vi "PQsetClientEncoding.vi"(8 "error in (no error)":errorcluster, 10 "encoding":string, 11 "conn":u32) -> (0 "error out":errorcluster, 2 "PQsetClientEncoding":i32)   [LabVIEW 2017, in "libpqlv.lvlib"]
uses:
  libpqlv.lvlib
  lib/libpq.dll
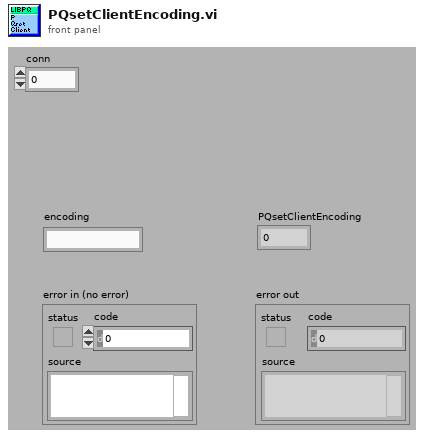
[diagram p1: front panel]
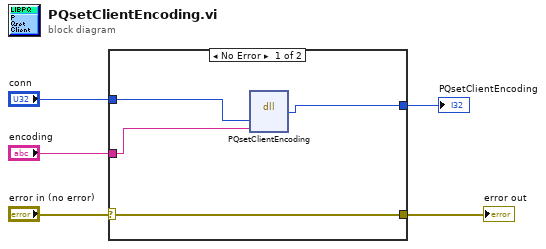
[diagram p0: block diagram]
diagram:
  n1 = case shown="No Error" "error in (no error)" {
    selector: "error in (no error)" -> [w9 w10]
    tunnel: [w9 w10] -> w4
    tunnel: [w8 _] -> w3
    tunnel: "encoding" -> [w7 _]
    tunnel: "conn" -> [w6 _]
    frame No Error {
      n2 = dll-call lib="D:/Users/erics/Documents/active/DAQ/PostgreSQL2LabVIEW/libpqlv/lib/libpq.*" fn="PQsetClientEncoding"("conn"=w6, "encoding"=w7) -> ("PQsetClientEncoding"=w8:i32)  [unwired: 5 in, 2 out]
    }
    frame Error {
    }
  }
  "PQsetClientEncoding" <- w3
  "error out" <- w4
